vi "Write HttpHeaders.vi"(8 "error in (no error)":errorcluster, 10 "HttpHeaders":refnum<class "HttpHeaders_Request.lvclass">, 11 "HttpRequestMessage in":refnum<class "HttpRequestMessage.lvclass">) -> (0 "error out":errorcluster, 3 "HttpRequestMessage out":refnum<class "HttpRequestMessage.lvclass">)   [LabVIEW 2018]
uses:
  HttpRequestMessage.lvclass
  HttpHeaders_Request/HttpHeaders_Request.lvclass
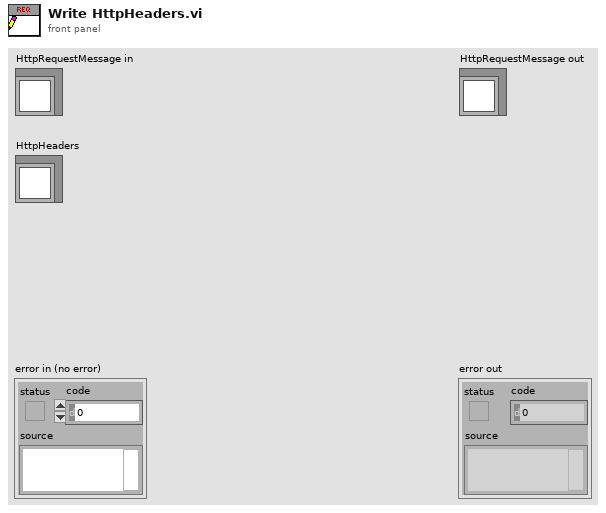
[diagram p1: front panel]
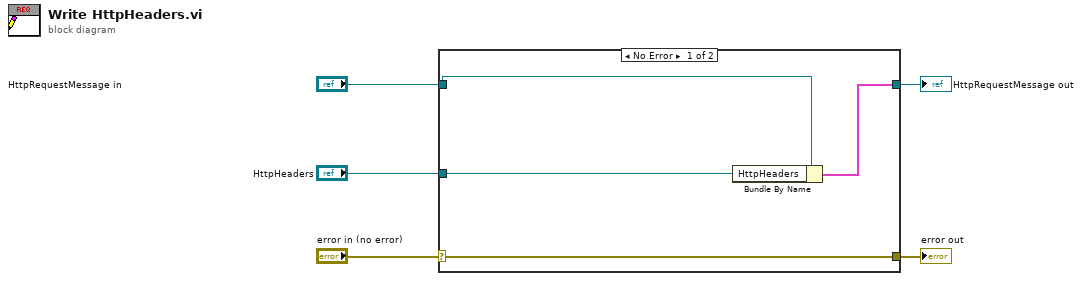
[diagram p0: block diagram]
diagram:
  n1 = case shown="No Error" "error in (no error)" {
    selector: "error in (no error)" -> [w9 w10]
    tunnel: [w9 w10] -> w4
    tunnel: [w7 w11] -> w2
    tunnel: "HttpRequestMessage in" -> [w8 w11]
    tunnel: "HttpHeaders" -> [w6 _]
    frame No Error {
      n2 = Bundle By Name(cluster=w8, "HttpHeaders"=w6) -> (w7:cluster{})
    }
    frame Error {
    }
  }
  "error out" <- w4
  "HttpRequestMessage out" <- w2
